vi "Internal Message Loop.vi"(8 "error in (no error)":errorcluster, 11 "WAMP Client in":refnum<class "WAMP Client.lvclass">) -> (0 "error out":errorcluster, 3 "WAMP Client out":refnum<class "WAMP Client.lvclass">)   [LabVIEW 2020, in "wamplv.lvlib" / "WAMP Client.lvclass"]
uses:
  WAMP Client.lvclass
  WAMP Client.lvclass/WAMP Client.ctl
  TypeDef/Message Loop Shift Reg Data.ctl
  TypeDef/REGISTER Request Data.ctl
  TypeDef/Success or error.ctl
  API/TypeDefs/Combined error.ctl
  API/TypeDefs/WAMP error.ctl
  TypeDef/Publish Requests Map.ctl
  TypeDef/PUBLISH Request Data.ctl
  TypeDef/PUBLISH result.ctl
  TypeDef/Endpoint Data.ctl
  TypeDef/CALL Request Map.ctl
  TypeDef/CALL Request Data.ctl
  API/TypeDefs/RESULT payload.ctl
  TypeDef/SUBSCRIBE Requests Map.ctl
  TypeDef/SUBSCRIBE Request Data.ctl
  TypeDef/Subscribe Result.ctl
  TypeDef/EVENT payload.ctl
  TypeDef/Subscriptions Map.ctl
  TypeDef/Subscription Details.ctl
  TypeDef/Unsubscribe Requests Map.ctl
  TypeDef/UNSUBSCRIBE Request Data.ctl
  TypeDef/UNSUBSCRIBE Result.ctl
  TypeDef/Unregister requests map.ctl
  TypeDef/Unregister request.ctl
  TypeDef/WAMP Received Message.ctl
  TypeDef/WAMP Message Codes.ctl
  TypeDef/GOODBYE Request Data.ctl
  TypeDef/Termination Reason Enum.ctl
  0ad20a80-b884-3f82-8ee8-d8e935c3ee3f.vi
  08e67e80-cc16-3fac-40e3-ebe0e858da3f.vi
  SubVIs/Get Subscription ID of topic.vi
  SubVIs/Handlers/Handle UNSUBSCRIBED.vi/73a204a7-fc9f-47f9-93b3-f48d89583bd3.vi
  SubVIs/WAMP message creators/Create PUBLISH msg.vi
  SubVIs/WAMP message creators/Create CALL msg.vi
  SubVIs/Handlers/Handle RESULT.vi/fe43fee3-e626-436a-9df9-4c595b512d78.vi
  SubVIs/Handlers/Handle UNREGISTERED.vi/270ddf32-b247-4482-b6bc-5475b82892bf.vi
  SubVIs/WAMP message creators/Create YIELD msg.vi
  SubVIs/Check Empty JSON String.vi
  SubVIs/Check Empty JSON Array.vi
  SubVIs/WAMP to LV error.vi
  <vilib>/Utility/error.llb/Error Cluster From Error Code.vi
  <vilib>/JDP Science/JSONtext/Set Item.vi
  SubVIs/Get Registration ID of endpoint.vi
  SubVIs/Increment request ID.vi
  SubVIs/WAMP message creators/Create UNREGISTER msg.vi
  Private/Invocation Request ID/Create New.vi
  <vilib>/JDP Science/JSONtext/LVClass Serializer/JSONtext LVClass Serializer.lvclass
  Private/Invocation Request ID/Invocation Request ID.lvclass
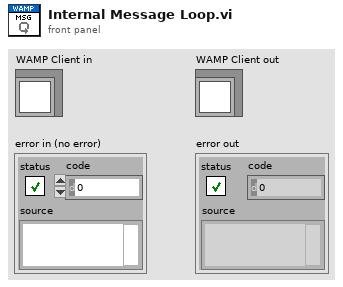
[diagram p1: front panel]
types:
  T1 = typedef "wamplv.lvlib/WAMP Client.lvclass/Message Loop Shift Reg Data.ctl" = cluster{"Last Request ID":u64, "Register Requests":map{u64, T2}, "Publish Requests":T3, "Endpoints Map":map{u64, T5}, "Call Requests":T6, "Subscription Requests":T8, "Subscriptions":T10, "Unsubscribe Requests":T12, "Random Request IDs":u64[], "Unregister requests map":T14}
  T2 = typedef "wamplv.lvlib/WAMP Client.lvclass/REGISTER Request Data.ctl" = cluster{"Procedure URI":string, "Options":string, "REGISTER result notifier":refnum<notifier>}
  T3 = typedef "wamplv.lvlib/WAMP Client.lvclass/Publish Requests Map.ctl" = map{u64, T4}
  T4 = typedef "wamplv.lvlib/WAMP Client.lvclass/PUBLISH Request Data.ctl" = cluster{"Topic URI":string, "Arguments":string, "ArgumentsKw":string, "Request Acknowledgement":bool, "Options":string, "Publish result notifier":refnum<notifier>}
  T5 = typedef "wamplv.lvlib/WAMP Client.lvclass/Endpoint Data.ctl" = cluster{"Procedure URI":string}
  T6 = typedef "wamplv.lvlib/WAMP Client.lvclass/CALL Request Map.ctl" = map{u64, T7}
  T7 = typedef "wamplv.lvlib/WAMP Client.lvclass/CALL Request Data.ctl" = cluster{"Topic URI":string, "Arguments":string, "ArgumentsKw":string, "Options":string, "Call result":refnum<notifier>}
  T8 = typedef "wamplv.lvlib/WAMP Client.lvclass/SUBSCRIBE Requests Map.ctl" = map{u64, T9}
  T9 = typedef "wamplv.lvlib/WAMP Client.lvclass/SUBSCRIBE Request Data.ctl" = cluster{"Topic":string, "Subscribe result notifer":refnum<notifier>, "Options":string}
  T10 = typedef "wamplv.lvlib/WAMP Client.lvclass/Subscriptions Map.ctl" = map{u64, T11}
  T11 = typedef "wamplv.lvlib/WAMP Client.lvclass/Subscription Details.ctl" = cluster{"Subscription ID":u64, "Topic":string, "Publication Received Event":refnum<user-event>}
  T12 = typedef "wamplv.lvlib/WAMP Client.lvclass/Unsubscribe Requests Map.ctl" = map{u64, T13}
  T13 = typedef "wamplv.lvlib/WAMP Client.lvclass/UNSUBSCRIBE Request Data.ctl" = cluster{"Topic":string, "Unsubscrube result notifier":refnum<notifier>, "Options":string}
  T14 = typedef "wamplv.lvlib/WAMP Client.lvclass/Unregister requests map.ctl" = map{u64, T15}
  T15 = typedef "wamplv.lvlib/WAMP Client.lvclass/Unregister request.ctl" = cluster{"URI":string, "Unregister result notifier":refnum<notifier>, "Options":string}
  T16 = typedef "wamplv.lvlib/WAMP Client.lvclass/WAMP Received Message.ctl" = cluster{"Message JSON":string[], "Message Codes":T17}
  T17 = typedef "wamplv.lvlib/WAMP Client.lvclass/WAMP Message Codes.ctl" = u16
  T18 = typedef "wamplv.lvlib/WAMP Client.lvclass/GOODBYE Request Data.ctl" = cluster{"Error URI":string, "Message":string}
  T19 = typedef "wamplv.lvlib/WAMP Client.lvclass/Termination Reason Enum.ctl" = enum16{"Goodbye Received", "Abort Received", "Send Goodbye", "Send Abort", "Read Loop Failure", "Write Loop Failure", "Message Loop Failure"}
  T20 = typedef "wamplv.lvlib/WAMP Client.lvclass/Internal Message.ctl" = cluster{"Internal Message Type":T21, "Variant":variant}
  T21 = typedef "wamplv.lvlib/WAMP Client.lvclass/Internal Message Type.ctl" = enum16{"Subscribe", "Handle Subscribed", "Handle Event", "Unsubscribe", "Handle Unsubscribed", "Publish", "Handled Published", "Goodbye", "Handle Goodbye", "Call", "Handle Result", "Register", "Handle Registered", "Unregister", "Handle Unregistered", "Handle Invocation", "Yield", "Error"}
  T22 = typedef "wamplv.lvlib/WAMP Client.lvclass/YIELD request data.ctl" = cluster{"Invocation Request ID":u64, "Arguments":string, "ArgumentsKw":string, "Options":string}
  T23 = typedef "wamplv.lvlib/WAMP Client.lvclass/Error Request.ctl" = cluster{"WAMP Error":T24, "Message Type":T17, "Request ID":u64}
  T24 = typedef "wamplv.lvlib/WAMP Client.lvclass/WAMP error.ctl" = cluster{"Details":string, "ArgumentKw Payload":string, "Error?":bool, "Error URI":string, "Arguments Payload":string}
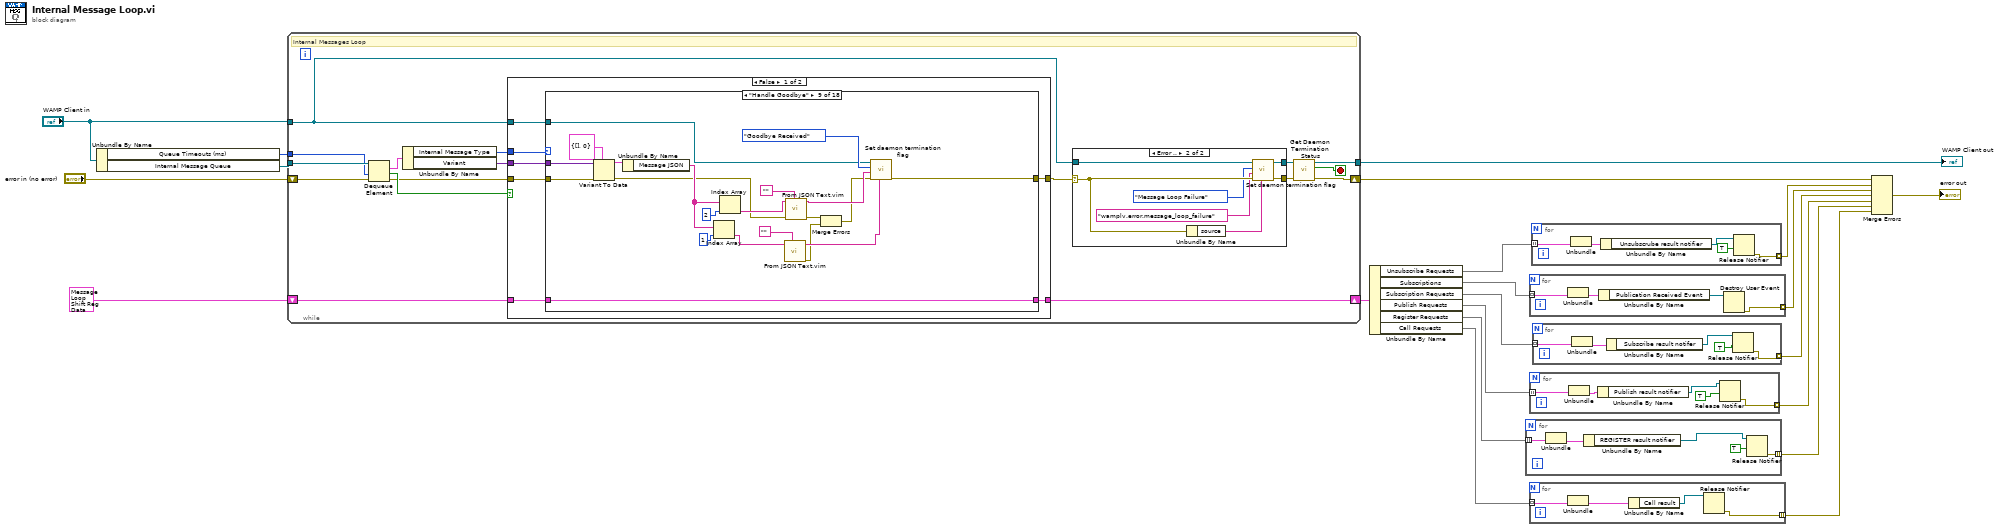
[diagram p0: block diagram]
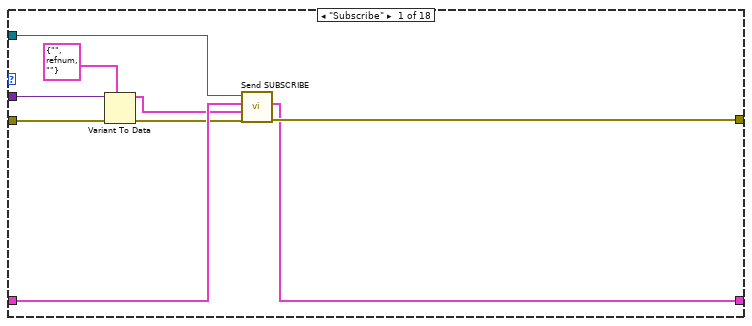
[diagram p2: hidden frame]
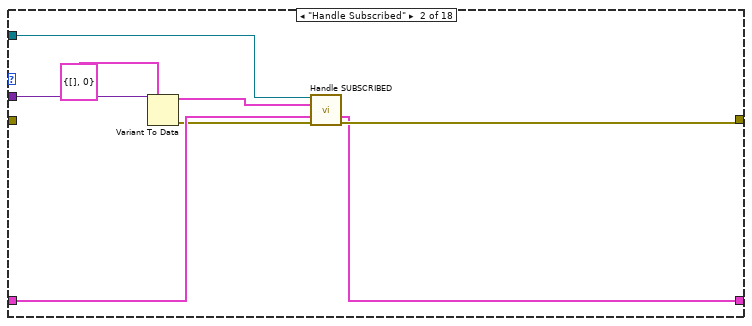
[diagram p3: hidden frame]
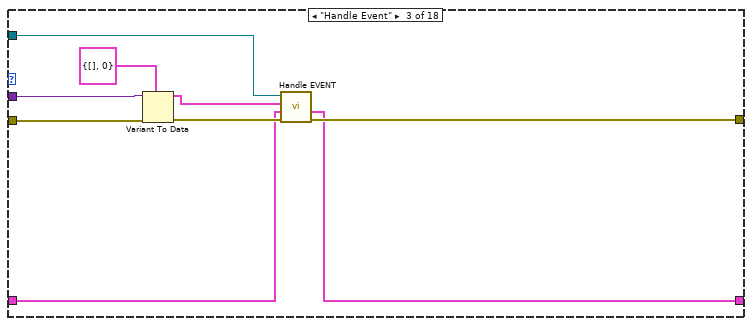
[diagram p4: hidden frame]
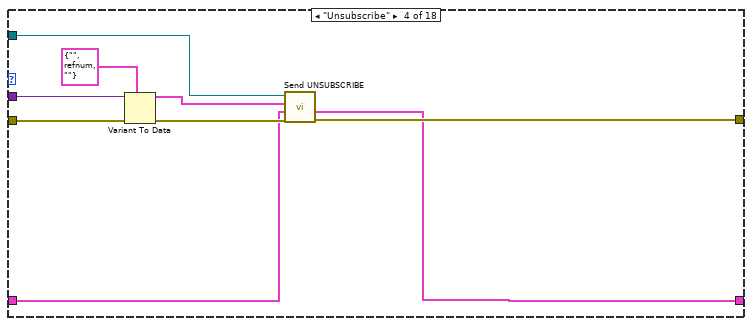
[diagram p5: hidden frame]
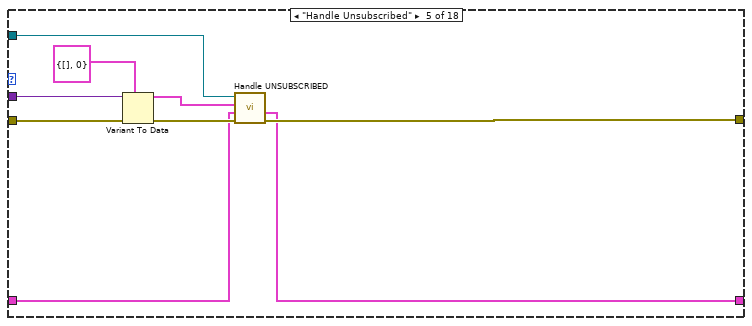
[diagram p6: hidden frame]
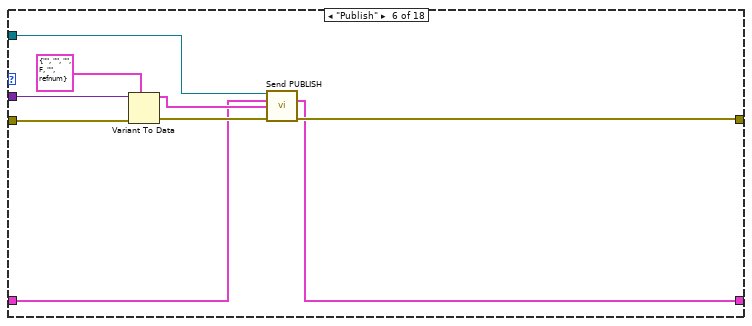
[diagram p7: hidden frame]
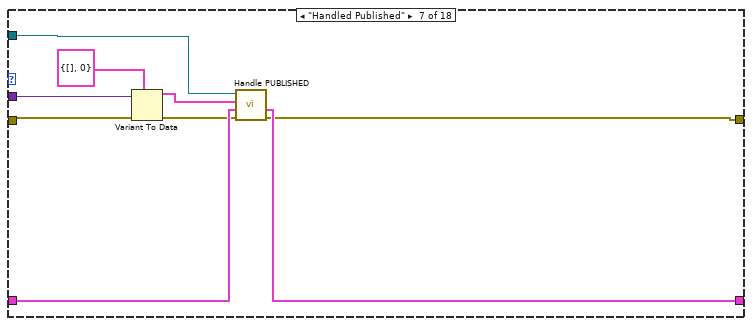
[diagram p8: hidden frame]
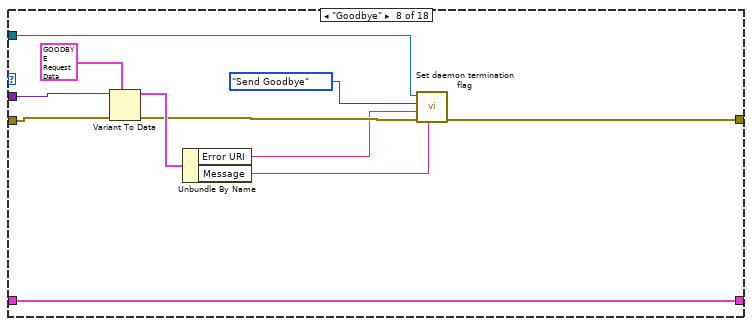
[diagram p9: hidden frame]
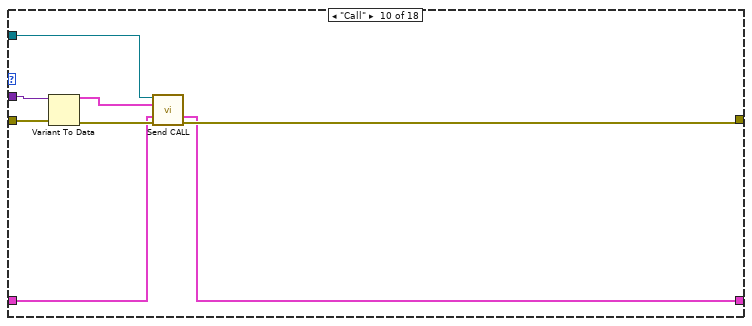
[diagram p10: hidden frame]
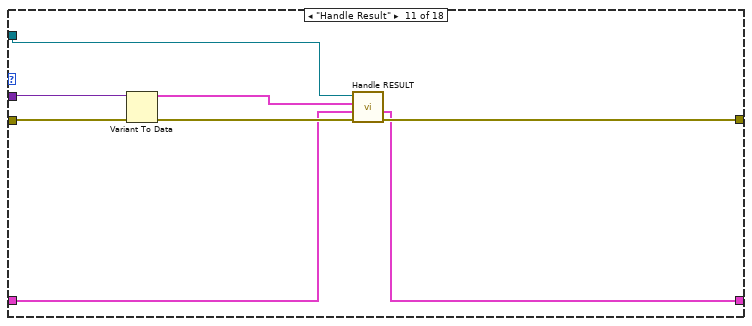
[diagram p11: hidden frame]
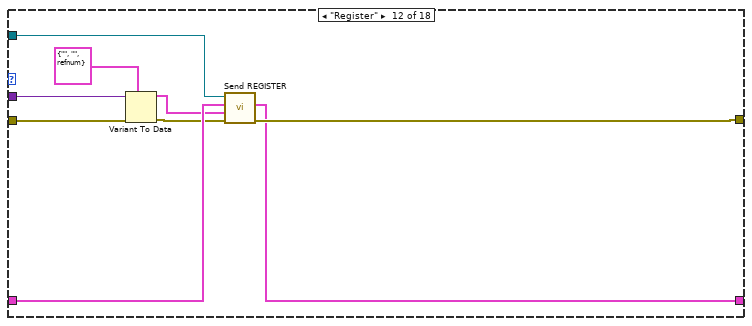
[diagram p12: hidden frame]
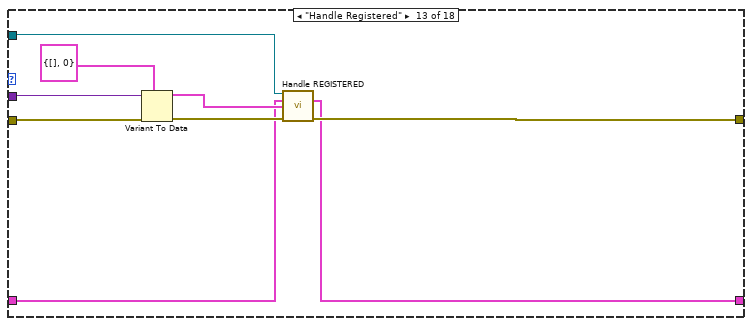
[diagram p13: hidden frame]
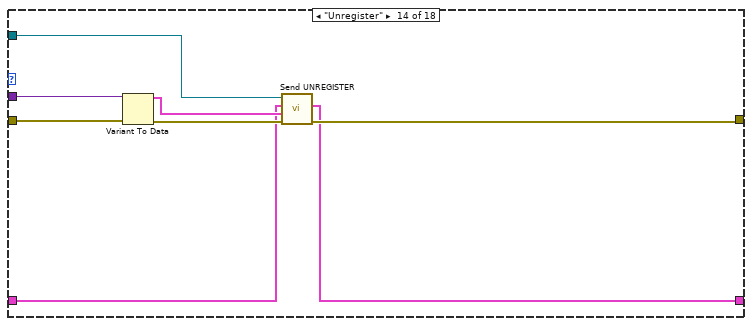
[diagram p14: hidden frame]
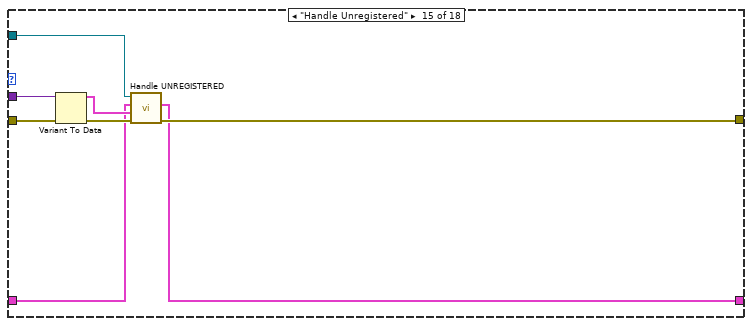
[diagram p15: hidden frame]
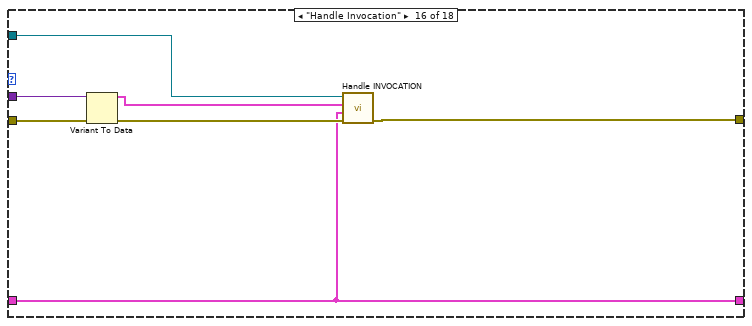
[diagram p16: hidden frame]
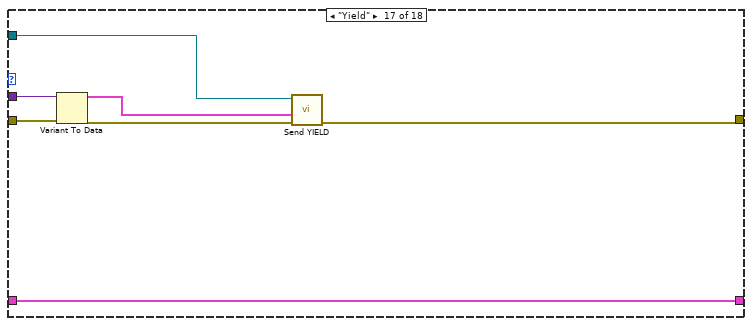
[diagram p17: hidden frame]
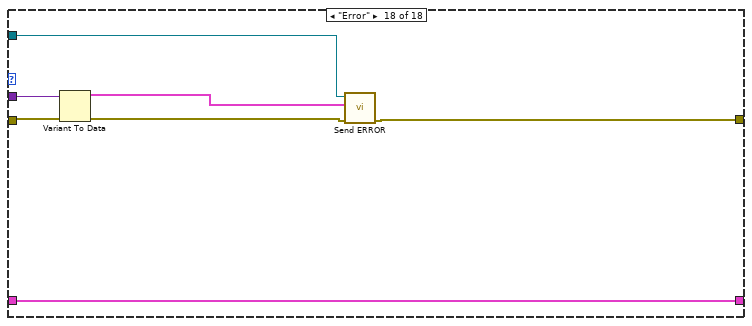
[diagram p18: hidden frame]
diagram:
  n1 = Unbundle By Name("WAMP Client in") -> ("Queue Timeouts (ms)"=w3:i32, "Internal Message Queue"=w21:refnum<queue>)
  n2 = while {
    tunnel: w21 -> [w38]
    tunnel: "WAMP Client in" -> [w30]
    shift-right: [w32] -> w18
    shift-left: "error in (no error)" -> [w37]
    shift-right: [w29] -> w16
    shift-left: T1 {"Last Request ID"=0, "Register Requests"={}, "Publish Requests"={}, "Endpoints Map"={}, "Call Requests"={}, "Subscription Requests"={}, "Subscriptions"={}, "Unsubscribe Requests"={}, "Random Request IDs"=[], "Unregister requests map"={}} ("Message Loop Shift Register Data") -> [w35]
    tunnel: w3 -> [w28]
    tunnel: [w27] -> w1
    stop <- w31 stop-if-true
    # "Internal Messages Loop"
    n3 = Dequeue Element(queue=w38, timeout in ms (-1)=w28, error in (no error)=w37) -> (element=w26:T20, timed out?=w23:bool, error out=w22:errorcluster)  [unwired: 1 out]
    n4 = Unbundle By Name(w26) -> ("Internal Message Type"=w25:T21, "Variant"=w24:variant)
    n5 = case shown="False" w23 {
      tunnel: w25 -> [w45 _]
      tunnel: w24 -> [w44 _]
      tunnel: w30 -> [w43 _]
      tunnel: w22 -> [w42 w212]
      tunnel: [w41 w212] -> w36
      tunnel: w35 -> [w40 w211]
      tunnel: [w39 w211] -> w29
      frame False {
        n6 = case shown="\"Handle Goodbye\"" w45 {
          tunnel: w44 -> [w54 w61 w70 w80 w89 w98 w106 w118 w137 w147 w154 w163 w173 w181 w187 w195 w203 w206]
          tunnel: w43 -> [w52 w62 w71 w79 w87 w93 w103 w112 w130 w145 w155 w161 w169 w177 w185 w196 w199 w209]
          tunnel: w42 -> [w47 _ w68 w76 w85 w95 w104 w116 w138 w146 w153 w162 w172 w180 w189 w194 w202 w207]
          tunnel: [w51 w56 w67 w74 w82 w91 w100 w114 w139 w141 w151 w160 w167 w176 w183 w192 w198 w210] -> w41
          tunnel: w40 -> [w50 w59 w64 w73 w83 w92 w102 w108 w129 w142 w149 w158 w166 w175 w184 w190 w197 w204]
          tunnel: [w46 w55 w63 w72 w81 w90 w101 w108 w129 w140 w148 w159 w165 w174 w182 w190 w197 w204] -> w39
          frame "Subscribe" {
            n7 = Variant To Data(error in=w47, type=T9 {"Topic"="", "Subscribe result notifer"=refnum, "Options"=""} ("Cluster"), Variant=w54) -> (data=w49:T9, error out=w48:errorcluster)
            n8 = call "Send SUBSCRIBE.vi"("error in"=w48, "Subscription Request"=w49, "Message Loop Data (in)"=w50, "WAMP Client in"=w52) -> ("error out"=w51:errorcluster, "Message Loop Data (out)"=w46:T1)  [unwired: 5 in, 1 out]
          }
          frame "Handle Subscribed" {
            n9 = Variant To Data(type=T16 {"Message JSON"=[], "Message Codes"=0} ("Cluster"), Variant=w61) -> (data=w58:T16, error out=w57:errorcluster)  [unwired: 1 in]
            n10 = call "Handle SUBSCRIBED.vi"("reference"=w62, "WAMP Message"=w58, "Message Loop data (in)"=w59, "error in (no error)"=w57) -> ("Message Loop Data (out)"=w55:T1, "error out"=w56:errorcluster)  [unwired: 9 in, 1 out]
          }
          frame "Handle Event" {
            n11 = Variant To Data(error in=w68, type=T16 {"Message JSON"=[], "Message Codes"=0} ("Cluster"), Variant=w70) -> (data=w65:T16, error out=w66:errorcluster)
            n12 = call "Handle EVENT.vi"("error in (no error)"=w66, "Message Loop Data (in)"=w64, "Cluster"=w65, "reference"=w71) -> ("error out"=w67:errorcluster, "Message Loop Data (out)"=w63:T1)  [unwired: 5 in, 1 out]
          }
          frame "Unsubscribe" {
            n13 = Variant To Data(error in=w76, type=T13 {"Topic"="", "Unsubscrube result notifier"=refnum, "Options"=""} ("Cluster"), Variant=w80) -> (data=w78:T13, error out=w75:errorcluster)
            n14 = call "Send UNSUBSCRIBE.vi"("error in (no error)"=w75, "Message loop data (in)"=w73, "Unsubscribe Request Data"=w78, "WAMP Client in"=w79) -> ("error out"=w74:errorcluster, "Message loop data (out)"=w72:T1)  [unwired: 5 in, 1 out]
          }
          frame "Handle Unsubscribed" {
            n15 = Variant To Data(error in=w85, type=T16 {"Message JSON"=[], "Message Codes"=0} ("Cluster"), Variant=w89) -> (data=w86:T16, error out=w84:errorcluster)
            n16 = call "Handle UNSUBSCRIBED.vi"("error in (no error)"=w84, "Message Loop data (in)"=w83, "WAMP Message"=w86, "reference"=w87) -> ("error out"=w82:errorcluster, "Message Loop Data (Out)"=w81:T1)  [unwired: 5 in, 1 out]
          }
          frame "Publish" {
            n17 = Variant To Data(error in=w95, type=T4 {"Topic URI"="", "Arguments"="", "ArgumentsKw"="", "Request Acknowledgement"=FALSE, "Options"="", "Publish result notifier"=refnum} ("Cluster"), Variant=w98) -> (data=w96:T4, error out=w94:errorcluster)
            n18 = call "Send PUBLISH.vi"("WAMP Client in"=w93, "Message Loop Shift Register Data (In)"=w92, "Publish Request Data"=w96, "error in (no error)"=w94) -> ("Message Loop Shift Register Data (Out)"=w90:T1, "error out"=w91:errorcluster)  [unwired: 9 in, 1 out]
          }
          frame "Handled Published" {
            n19 = Variant To Data(error in=w104, type=T16 {"Message JSON"=[], "Message Codes"=0} ("Cluster"), Variant=w106) -> (data=w105:T16, error out=w99:errorcluster)
            n20 = call "Handle PUBLISHED.vi"("error in (no error)"=w99, "Message Loop data (in)"=w102, "WAMP Message"=w105, "reference"=w103) -> ("error out"=w100:errorcluster, "Message Loop data (out)"=w101:T1)  [unwired: 5 in, 1 out]
          }
          frame "Goodbye" {
            n21 = Variant To Data(error in=w116, type=T18 {"Error URI"="wamp.error.protocol_violation", "Message"="wamp.close.shut_down"} ("Goodbye Request"), Variant=w118) -> (data=w115:T18, error out=w113:errorcluster)
            n22 = Unbundle By Name(w115) -> ("Error URI"=w110:string, "Message"=w109:string)
            n23 = call "Set daemon termination flag.vi"("Message"=w109, "error in (no error)"=w113, "Reason URI"=w110, "Reason"=Termination_Reason_Enum."Send Goodbye" ("Termination Reason"), "WAMP Client (in)"=w112) -> ("error out"=w114:errorcluster)  [unwired: 5 in, 1 out]
          }
          frame "Handle Goodbye" {
            n24 = Variant To Data(error in=w138, type=T16 {"Message JSON"=[], "Message Codes"=0} ("Cluster"), Variant=w137) -> (data=w135:T16, error out=w122:errorcluster)
            n25 = Unbundle By Name(w135) -> ("Message JSON"=w132:string[])
            n26 = Index Array(array=w132, index=1) -> (element=w124:string)
            n27 = Index Array(array=w132, index=2) -> (element=w128:string)
            n28 = call "From JSON Text.vim"("Data Type and Default Value"="" ("Empty String Constant"), "JSON"=w124) -> ("error out"=w119:errorcluster, "Data out"=w125:string)  [unwired: 8 in]
            n29 = call "From JSON Text.vim"("Data Type and Default Value"="" ("Empty String Constant"), "error in (no error)"=w122, "JSON"=w128) -> ("error out"=w120:errorcluster, "Data out"=w126:string)  [unwired: 7 in]
            n30 = Merge Errors(w120, w119) -> (w121:errorcluster)
            n31 = call "Set daemon termination flag.vi"("Message"=w125, "error in (no error)"=w121, "Reason URI"=w126, "Reason"=Termination_Reason_Enum."Goodbye Received" ("Termination Reason"), "WAMP Client (in)"=w130) -> ("error out"=w139:errorcluster)  [unwired: 5 in, 1 out]
          }
          frame "Call" {
            n32 = Variant To Data(error in=w146, Variant=w147) -> (data=w143:T7, error out=w144:errorcluster)  [unwired: 1 in]
            n33 = call "Send CALL.vi"("WAMP Client in"=w145, "Call Request"=w143, "Message Loop Shift Register Data"=w142, "error in"=w144) -> ("Message Loop Shift Register Data (out)"=w140:T1, "error out"=w141:errorcluster)  [unwired: 9 in, 1 out]
          }
          frame "Handle Result" {
            n34 = Variant To Data(error in=w153, Variant=w154) -> (data=w152:T16, error out=w150:errorcluster)  [unwired: 1 in]
            n35 = call "Handle RESULT.vi"("error in (no error)"=w150, "Message Loop Shift Register Data"=w149, "WAMP Message"=w152, "reference"=w155) -> ("error out"=w151:errorcluster, "Message Loop Shift Register Data (out)"=w148:T1)  [unwired: 5 in, 1 out]
          }
          frame "Register" {
            n36 = Variant To Data(error in=w162, type=T2 {"Procedure URI"="", "Options"="", "REGISTER result notifier"=refnum} ("REGISTER request data"), Variant=w163) -> (data=w157:T2, error out=w156:errorcluster)
            n37 = call "Send REGISTER.vi"("error in (no error)"=w156, "REGISTER request data"=w157, "Message Loop Shift Register Data in"=w158, "WAMP Client in"=w161) -> ("error out"=w160:errorcluster, "Message Loop Shift Register Data out"=w159:T1)  [unwired: 5 in, 1 out]
          }
          frame "Handle Registered" {
            n38 = Variant To Data(error in=w172, type=T16 {"Message JSON"=[], "Message Codes"=0} ("Cluster"), Variant=w173) -> (data=w171:T16, error out=w168:errorcluster)
            n39 = call "Handle REGISTERED.vi"("WAMP Client in"=w169, "Message Loop Shift Register Data"=w166, "WAMP Message"=w171, "error in (no error)"=w168) -> ("output cluster"=w165:T1, "error out"=w167:errorcluster)  [unwired: 9 in, 1 out]
          }
          frame "Unregister" {
            n40 = Variant To Data(error in=w180, Variant=w181) -> (data=w179:T15, error out=w178:errorcluster)  [unwired: 1 in]
            n41 = call "Send UNREGISTER.vi"("error in (no error)"=w178, "Unregister Request"=w179, "Message loop data (in)"=w175, "WAMP Client in"=w177) -> ("error out"=w176:errorcluster, "Message loop data (out)"=w174:T1)  [unwired: 5 in, 1 out]
          }
          frame "Handle Unregistered" {
            n42 = Variant To Data(error in=w189, Variant=w187) -> (data=w186:T16, error out=w188:errorcluster)  [unwired: 1 in]
            n43 = call "Handle UNREGISTERED.vi"("error in (no error)"=w188, "WAMP Message"=w186, "Message loop data (in)"=w184, "reference"=w185) -> ("error out"=w183:errorcluster, "Message Loop Data (Out)"=w182:T1)  [unwired: 5 in, 1 out]
          }
          frame "Handle Invocation" {
            n44 = Variant To Data(error in=w194, Variant=w195) -> (data=w191:T16, error out=w193:errorcluster)  [unwired: 1 in]
            n45 = call "Handle INVOCATION.vi"("error in (no error)"=w193, "Message Loop Shift Register Data"=w190, "Cluster"=w191, "reference"=w196) -> ("error out"=w192:errorcluster)  [unwired: 6 in, 1 out]
          }
          frame "Yield" {
            n46 = Variant To Data(error in=w202, Variant=w203) -> (data=w201:T22, error out=w200:errorcluster)  [unwired: 1 in]
            n47 = call "Send YIELD.vi"("error in (no error)"=w200, "Yield request"=w201, "WAMP Client in"=w199) -> ("error out"=w198:errorcluster)  [unwired: 7 in, 1 out]
          }
          frame "Error" {
            n48 = Variant To Data(error in=w207, Variant=w206) -> (data=w205:T23, error out=w208:errorcluster)  [unwired: 1 in]
            n49 = call-dynamic "Send ERROR.vi"("error in (no error)"=w208, "Error Request"=w205, "WAMP Client in"=w209) -> ("error out"=w210:errorcluster)  [unwired: 7 in, 1 out]
          }
        }
      }
      frame True {
        # "Time out, no internal messages"
      }
    }
    n50 = case shown="Error .." w36 {
      selector: w36 -> [w214 w220]
      tunnel: [w214 w221] -> w34
      tunnel: [w213 w219] -> w33
      tunnel: w30 -> [w213 w218]
      frame No Error {
      }
      frame Error {
        n51 = Unbundle By Name(w220) -> ("source"=w215:string)
        n52 = call "Set daemon termination flag.vi"("Message"=w215, "error in (no error)"=w220, "Reason URI"="wamplv.error.message_loop_failure" ("Error URI"), "Reason"=Termination_Reason_Enum."Message Loop Failure" ("Termination Reason"), "WAMP Client (in)"=w218) -> ("error out"=w221:errorcluster, "WAMP Client (out)"=w219:refnum<class "WAMP Client.lvclass">)  [unwired: 5 in]
      }
    }
    n53 = call "Get Daemon Termination Status.vi"("error in (no error)"=w34, "WAMP Client in"=w33) -> ("error out"=w32:errorcluster, "Terminate?"=w31:bool, "WAMP Client out"=w27:refnum<class "WAMP Client.lvclass">)  [unwired: 6 in, 1 out]
  }
  "WAMP Client out" <- w1
  n54 = Unbundle By Name(w16) -> ("Unsubscribe Requests"=w10:T12, "Subscriptions"=w11:T10, "Subscription Requests"=w12:T8, "Publish Requests"=w15:T3, "Register Requests"=w14:map{u64, T2}, "Call Requests"=w13:T6)
  n55 = for {
    tunnel: w14 -> [w226] mode=indexing
    tunnel: [w224] -> w5 mode=indexing
    n56 = Unbundle(w226) -> (w225:T2)  [unwired: 1 out]
    n57 = Unbundle By Name(w225) -> ("REGISTER result notifier"=w223:refnum<notifier>)
    n58 = Release Notifier(notifier=w223, force destroy? (F)=TRUE) -> (error out=w224:errorcluster)  [unwired: 1 in, 2 out]
  }
  n59 = for {
    tunnel: w11 -> [w230] mode=indexing
    tunnel: [w227] -> w8 mode=indexing
    n60 = Unbundle(w230) -> (w229:T11)  [unwired: 1 out]
    n61 = Unbundle By Name(w229) -> ("Publication Received Event"=w228:refnum<user-event>)
    n62 = Destroy User Event(user event=w228) -> (error out=w227:errorcluster)  [unwired: 1 in]
  }
  n63 = for {
    tunnel: w13 -> [w234] mode=indexing
    tunnel: [w231] -> w4 mode=indexing
    n64 = Unbundle(w234) -> (w233:T7)  [unwired: 1 out]
    n65 = Unbundle By Name(w233) -> ("Call result"=w232:refnum<notifier>)
    n66 = Release Notifier(notifier=w232) -> (error out=w231:errorcluster)  [unwired: 2 in, 2 out]
  }
  n67 = for {
    tunnel: w15 -> [w239] mode=indexing
    tunnel: [w237] -> w6 mode=indexing
    n68 = Unbundle(w239) -> (w238:T4)  [unwired: 1 out]
    n69 = Unbundle By Name(w238) -> ("Publish result notifier"=w236:refnum<notifier>)
    n70 = Release Notifier(notifier=w236, force destroy? (F)=TRUE) -> (error out=w237:errorcluster)  [unwired: 1 in, 2 out]
  }
  n71 = for {
    tunnel: w10 -> [w244] mode=indexing
    tunnel: [w242] -> w9 mode=indexing
    n72 = Unbundle(w244) -> (w243:T13)  [unwired: 1 out]
    n73 = Unbundle By Name(w243) -> ("Unsubscrube result notifier"=w241:refnum<notifier>)
    n74 = Release Notifier(notifier=w241, force destroy? (F)=TRUE) -> (error out=w242:errorcluster)  [unwired: 1 in, 2 out]
  }
  n75 = for {
    tunnel: w12 -> [w249] mode=indexing
    tunnel: [w245] -> w7 mode=indexing
    n76 = Unbundle(w249) -> (w248:T9)  [unwired: 1 out]
    n77 = Unbundle By Name(w248) -> ("Subscribe result notifer"=w247:refnum<notifier>)
    n78 = Release Notifier(notifier=w247, force destroy? (F)=TRUE) -> (error out=w245:errorcluster)  [unwired: 1 in, 2 out]
  }
  n79 = Merge Errors(w18, w9, w8, w7, w6, w5, w4) -> (→"error out":errorcluster)
